vi "Parse Navigation Results.vi"(9 "Cycle Time":dbl, 10 "Targeting Data In":T1, 11 "Target Data":string) -> (2 "Targeting Data Out":T1)   [LabVIEW 2017, in "VisionHW.lvlib"]
uses:
  VisionHW.lvlib
  TypeDef/CLUST_Targeting Data.ctl
  TypeDef/CLUST_Cube Data.ctl
  TypeDef/CLUST_Road Navigation Data.ctl
  <vilib>/regexp/Match Regular Expression.xnode
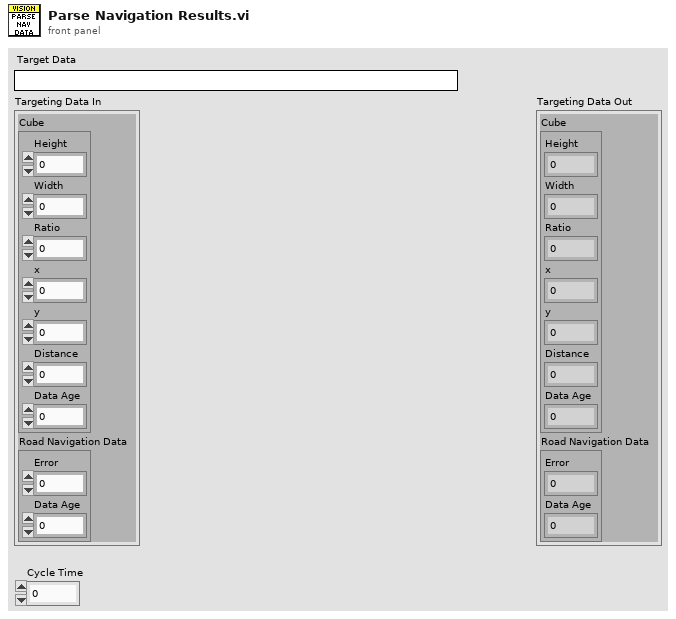
[diagram p1: front panel]
types:
  T1 = typedef "VisionHW.lvlib/CLUST_Targeting Data.ctl" = cluster{"Cube ":T2, "Road Navigation Data":T3}
  T2 = typedef "VisionHW.lvlib/CLUST_Cube Data.ctl" = cluster{"Height":dbl, "Width":dbl, "Ratio":dbl, "x":i32, "y":i32, "Distance ":i32, "Data Age":dbl}
  T3 = typedef "VisionHW.lvlib/CLUST_Road Navigation Data.ctl" = cluster{"Error":i32, "Data Age":dbl}
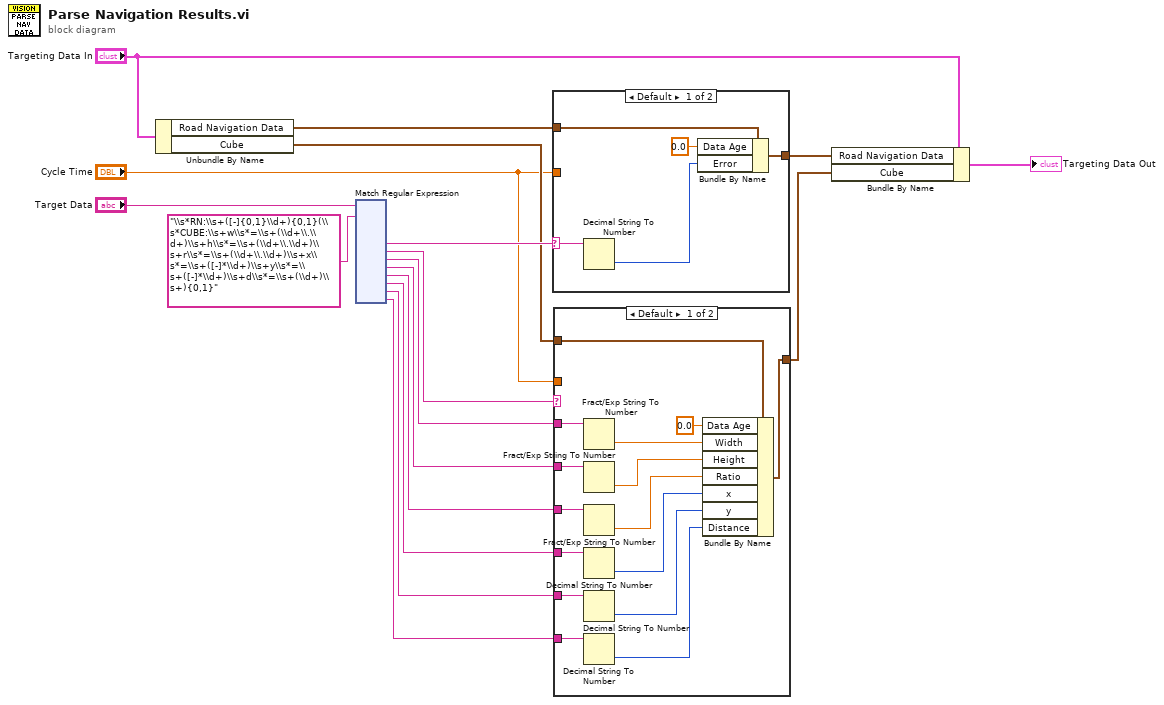
[diagram p0: block diagram]
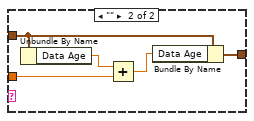
[diagram p2: hidden frame]
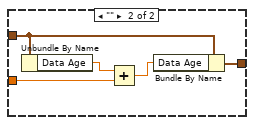
[diagram p3: hidden frame]
diagram:
  n1 = Unbundle By Name("Targeting Data In") -> ("Road Navigation Data"=w7:T3, "Cube"=w6:T2)
  n2 = xnode "Match Regular Expression"("input string"="Target Data", "regular expression"="\\s*RN:\\s+([-]{0,1}\\d+){0,1}(\\s*CUBE:\\s+w\\s*=\\s+(\\d+\\.\\d+)\\s+h\\s*=\\s+(\\d+\\.\\d+)\\s+r\\s*=\\s+(\\d+\\.\\d+)\\s+x\\s*=\\s+([-]*\\d+)\\s+y\\s*=\\s+([-]*\\d+)\\s+d\\s*=\\s+(\\d+)\\s+){0,1}") -> ("submatch 1"=w15:string, "submatch 2"=w14:string, "submatch 3"=w13:string, "submatch 4"=w12:string, "submatch 5"=w11:string, "submatch 6"=w10:string, "submatch 7"=w9:string, "submatch 8"=w8:string)  [unwired: 4 in, 5 out]
  n3 = case shown="Default" w15 {
    selector: w15 -> [w22 _]
    tunnel: w7 -> [w21 w26]
    tunnel: [w18 w27] -> w4
    tunnel: "Cycle Time" -> [_ w24]
    frame Default {
      n4 = Decimal String To Number(string=w22) -> (number=w20:i32)  [unwired: 2 in, 1 out]
      n5 = Bundle By Name(cluster=w21, "Data Age"=0.0, "Error"=w20) -> (w18:T3)
    }
    frame "" {
      n6 = Unbundle By Name(w26) -> ("Data Age"=w25:dbl)
      n7 = Add(x=w25, y=w24) -> (x+y=w23:dbl)
      n8 = Bundle By Name(cluster=w26, "Data Age"=w23) -> (w27:T3)
    }
  }
  n9 = case shown="Default" w14 {
    tunnel: w13 -> [w41 _]
    tunnel: w12 -> [w34 _]
    tunnel: w11 -> [w35 _]
    tunnel: w10 -> [w36 _]
    tunnel: w9 -> [w37 _]
    tunnel: w8 -> [w38 _]
    tunnel: w6 -> [w42 w47]
    tunnel: "Cycle Time" -> [_ w43]
    tunnel: [w28 w46] -> w2
    frame Default {
      n10 = Fract/Exp String To Number(string=w41) -> (number=w40:dbl)  [unwired: 3 in, 1 out]
      n11 = Fract/Exp String To Number(string=w34) -> (number=w29:dbl)  [unwired: 3 in, 1 out]
      n12 = Fract/Exp String To Number(string=w35) -> (number=w30:dbl)  [unwired: 3 in, 1 out]
      n13 = Decimal String To Number(string=w36) -> (number=w31:i32)  [unwired: 2 in, 1 out]
      n14 = Decimal String To Number(string=w37) -> (number=w32:i32)  [unwired: 2 in, 1 out]
      n15 = Decimal String To Number(string=w38) -> (number=w33:i32)  [unwired: 2 in, 1 out]
      n16 = Bundle By Name(cluster=w42, "Data Age"=0.0, "Width"=w40, "Height"=w29, "Ratio"=w30, "x"=w31, "y"=w32, "Distance"=w33) -> (w28:T2)
    }
    frame "" {
      n17 = Unbundle By Name(w47) -> ("Data Age"=w45:dbl)
      n18 = Add(x=w45, y=w43) -> (x+y=w44:dbl)
      n19 = Bundle By Name(cluster=w47, "Data Age"=w44) -> (w46:T2)
    }
  }
  n20 = Bundle By Name(cluster="Targeting Data In", "Road Navigation Data"=w4, "Cube"=w2) -> (→"Targeting Data Out":T1)
